vi "Log_Current_row_to_Execute.vi"(0 "Simulate/Run":T4, 1 "Message":string, 2 "Start of Multi Run Prog":bool, 3 "Traverse line in":T1 {"Carrier_2 Q (l/min)" format="%#.2f"; "Row Duration (mins)" format="%#.1f"; "Row No" min=0; "Trace Gas Concentration (%)" min=0.0 format="%#_4f"; "Carrier_1 Q (l/min)" format="%#.4f"; "Start X" format="%#.2f"; "Start Y" format="%#.2f"; "Start Z" format="%#.2f"; "End X" format="%#.2f"; "End Y" format="%#.2f"; "End Z" format="%#.2f"; "Tunnel Speed" format="%#.2f"; "Averaging time (mins)" min=0.0 format="%#.2f"}, 4 "Multi Run Log File":path) -> (9 "Traverse line Out":T1 {"Carrier_2 Q (l/min)" format="%#.2f"; "Row Duration (mins)" format="%#.1f"; "Row No" min=0; "Trace Gas Concentration (%)" min=0.0 format="%#_4f"; "Carrier_1 Q (l/min)" format="%#.4f"; "Start X" format="%#.2f"; "Start Y" format="%#.2f"; "Start Z" format="%#.2f"; "End X" format="%#.2f"; "End Y" format="%#.2f"; "End Z" format="%#.2f"; "Tunnel Speed" format="%#.2f"; "Averaging time (mins)" min=0.0 format="%#.2f"})   [LabVIEW 2020]
uses:
  Traverse_cluster.ctl
  Spacing.ctl
  Controls/Multi_run_mode.ctl
  Controls/User_Specific_mode.ctl
  Controls/Overhead.ctl
  Globals/Trav_pos_global.vi
panel:
  # "X                Y                   Z"
  # "X           Y          Z"
  # "Start"
  # "End"
  # "X           Y          Z"
  # "Start"
  # "End"
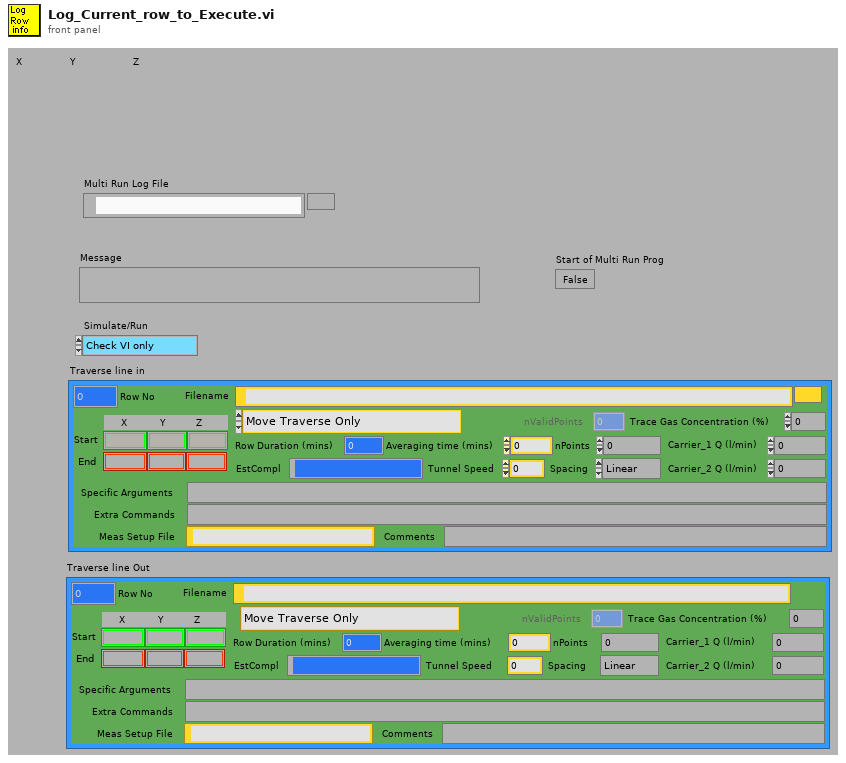
[diagram p1: front panel]
types:
  T1 = typedef "Traverse_cluster.ctl" = cluster{"Start X":sgl, "Start Y":sgl, "Start Z":sgl, "End X":sgl, "End Y":sgl, "End Z":sgl, "nPoints":i32, "Spacing":T2, "Filename":path, "Tunnel Speed":dbl, "Averaging time (mins)":dbl, "Extra Commands":string, "Carrier_1 Q (l/min)":dbl, "Carrier_2 Q (l/min)":dbl, "Trace Gas Concentration (%)":dbl, "Specific Arguments":string, "Comments":string, "Row No":i32, "Row Type Selector":T3, "EstCompl":string, "Row Duration (mins)":dbl, "nValidPoints":i32, "Meas Setup File":string}
  T2 = typedef "Spacing.ctl" = enum16{"Linear", "Log", "Gauss", "Specified", "N/A"}
  T3 = typedef "Multi_run_mode.ctl" = enum16{"Move Traverse Only", "Set Tunnel Speed Only", "Set Source Only", "Set Measurement Conditions", "Single Measurement", "Vertical Profile", "Lateral Profile", "Longitudinal Profile", "Multi-Axis Profile", "Explore Volume", "Auto Calibrate", "Meas Fast FID Bkgnd", "Check Beam Power", "Scanning Valve Measurement", "Run VI Named:", "Set ADAM Ch", "Wait (minutes)", "Send Message", "Synchronize With:", "Fall Back to this Row", "Turn Off Row Repeating", "Traverse 3D Volume", "Blank Row", "Jump to Fall Back Row"}
  T4 = typedef "User_Specific_mode.ctl" = enum16{"Check VI only", "Run VI"}
  T5 = enum16{"All Channel Names", "Valid Channel Names"}
  T6 = typedef "Overhead.ctl" = enum16{"Update total times", "Read Current Overhead", "Re Scale totals to 3 hrs", "Initialise totals to 3hr"}
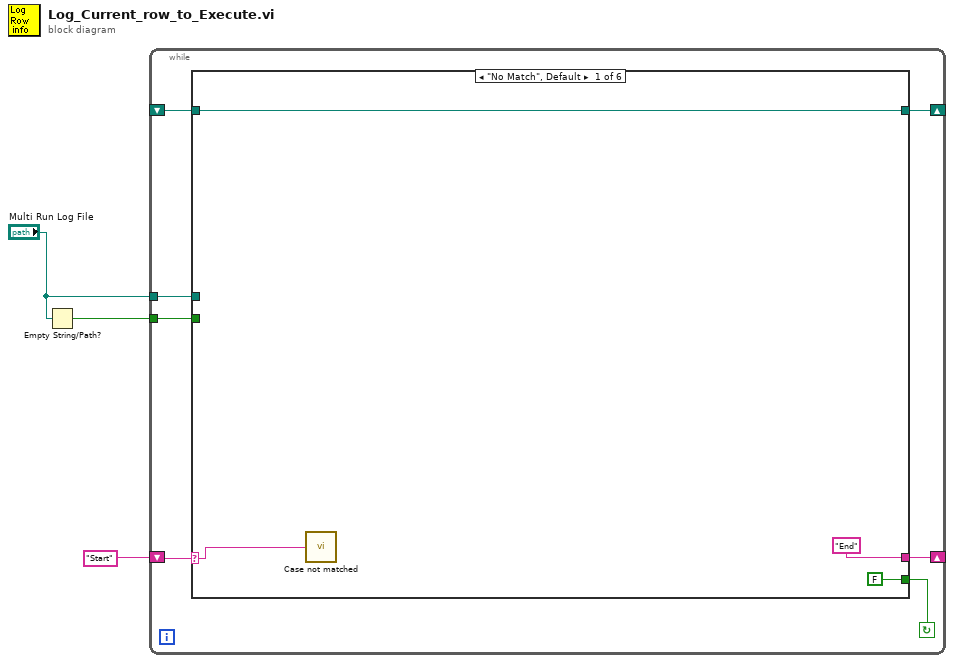
[diagram p0: block diagram]
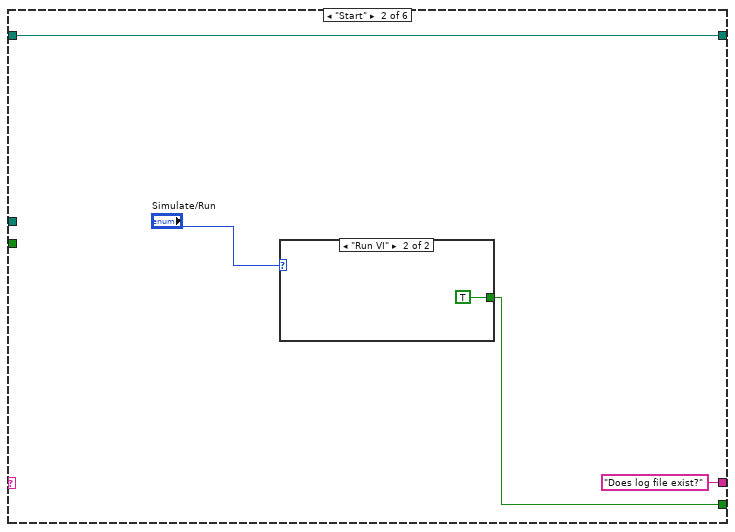
[diagram p2: hidden frame]
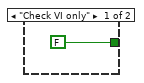
[diagram p3: hidden frame]
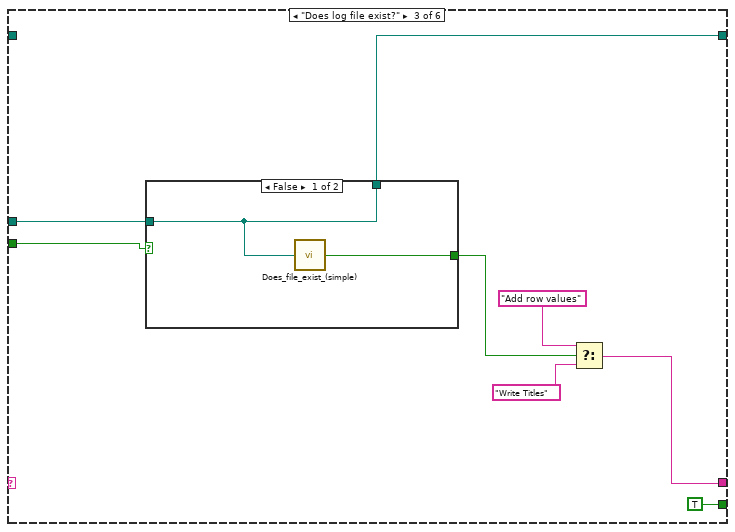
[diagram p4: hidden frame]
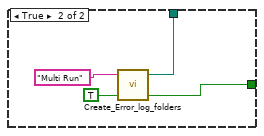
[diagram p5: hidden frame]
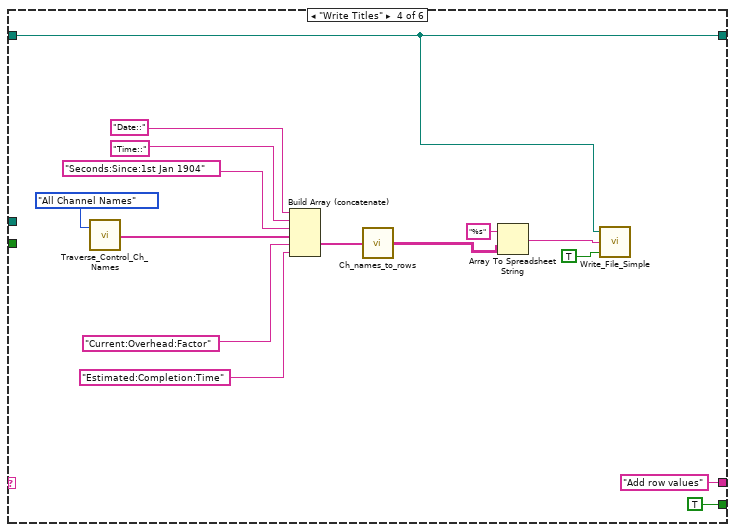
[diagram p6: hidden frame]
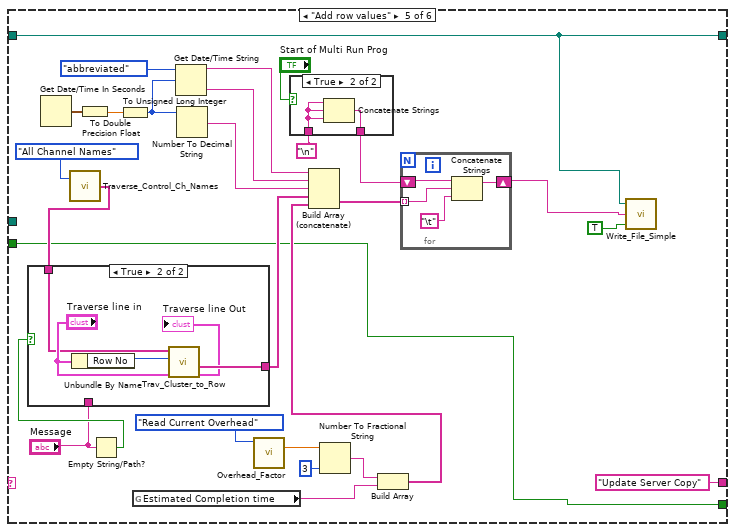
[diagram p7: hidden frame]
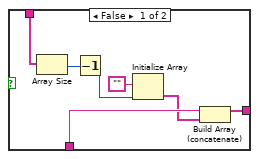
[diagram p9: hidden frame]
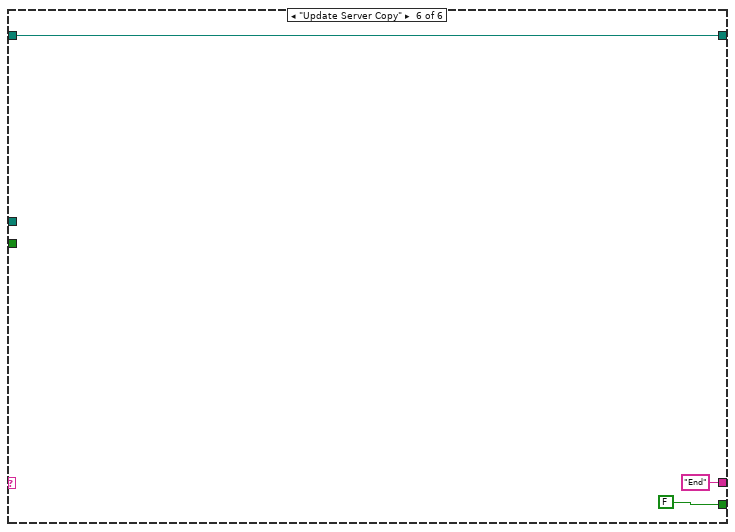
[diagram p10: hidden frame]
diagram:
  n1 = Empty String/Path?(string/path="Multi Run Log File") -> (empty?=w1:bool)
  n2 = while {
    shift-left: _ -> [w7]
    shift-right: [w8] -> _
    shift-left: "Start" -> [w6]
    shift-right: [w9] -> _
    tunnel: "Multi Run Log File" -> [w5]
    tunnel: w1 -> [w4]
    stop <- w10 continue-if-true
    n3 = case shown="\"No Match\", Default" w6 {
      selector: w6 -> [w11 _ _ _ _ _]
      tunnel: [FALSE ("T button?") w16 TRUE ("T button?") TRUE ("T button?") w53 FALSE] -> w10
      tunnel: ["End" "Does log file exist?" w28 "Add row values" "Update Server Copy" "End" ("f")] -> w9
      tunnel: [w12 w18 w26 w35 w50 w96] -> w8
      tunnel: w7 -> [w12 w18 _ w35 w50 w96]
      tunnel: w5 -> [_ _ w22 _ _ _]
      tunnel: w4 -> [_ _ w21 _ w53 _]
      frame "No Match", Default {
        n4 = call "Case not matched.vi"("Case Name not Matched"=w11) -> ()
      }
      frame "Start" {
        n5 = case shown="\"Run VI\"" "Simulate/Run" {
          tunnel: [FALSE TRUE] -> w16
          frame "Check VI only" {
          }
          frame "Run VI" {
          }
        }
      }
      frame "Does log file exist?" {
        n6 = case shown="False" w21 {
          tunnel: [w30 w34] -> w26
          tunnel: [w29 w32] -> w25
          tunnel: w22 -> [w30 _]
          frame False {
            n7 = call "Does_file_exist_(simple).vi"("Pathname"=w30) -> ("exists?"=w29:bool)
          }
          frame True {
            n8 = call "Create_Error_log_folders.vi"("Log Filename"="Multi Run" ("Input Element"), "Per Day Log File?"=TRUE) -> ("Local Log File"=w34:path, "exists?"=w32:bool)  [unwired: 4 in]
          }
        }
        n9 = Select(t="Add row values", s=w25, f="Write Titles") -> (s? t:f=w28:string)
      }
      frame "Write Titles" {
        n10 = call "Traverse_Control_Ch_Names.vi"("Mode"=T5."All Channel Names") -> ("Channel names"=w43:string[])  [unwired: 1 in]
        n11 = Build Array (concatenate)("Date::", "Time::", "Seconds:Since:1st Jan 1904", w43, "Current:Overhead:Factor", "Estimated:Completion:Time") -> (w40:string[])
        n12 = call "Ch_names_to_rows.vi"("Channel Names"=w40) -> ("3 Row names"=w39:string[][])
        n13 = Array To Spreadsheet String(array=w39, 3:"%s" ("format string")) -> (spreadsheet string=w36:string)  [unwired: 1 out]
        n14 = call "Write_File_Simple.vi"("append to file? (new file:F)"=TRUE, "character string"=w36, "file path"=w35) -> ()  [unwired: 2 out]
      }
      frame "Add row values" {
        n15 = Get Date/Time In Seconds() -> (seconds since 1Jan1904=w54:timestamp)
        n16 = call "Traverse_Control_Ch_Names.vi"("Mode"=T5."All Channel Names") -> ("Channel names"=w66:string[])  [unwired: 1 in]
        n17 = To Double Precision Float(number=w54) -> (double precision float=w75:dbl)
        n18 = Empty String/Path?(string/path="Message") -> (empty?=w68:bool)
        n19 = case shown="True" w68 {
          tunnel: w66 -> [w85 w89]
          tunnel: [w83 w88] -> w70
          tunnel: "Message" -> [w86 _]
          frame False {
            n20 = Array Size(array=w85) -> (size(s)=w82:i32)
            n21 = Decrement(x=w82) -> (x-1=w81:i32)
            n22 = Initialize Array("", w81) -> (w80:string[])
            n23 = Build Array (concatenate)(w86, w80) -> (w83:string[])
          }
          frame True {
            n24 = Unbundle By Name("Traverse line in") -> ("Row No"=w91:i32)
            n25 = call "Trav_Cluster_to_Row.vi"("Traverse line in"="Traverse line in", "Row Number"=w91, "Channel names"=w89) -> ("Traverse line Out"=→"Traverse line Out":T1, "Channel Values Out"=w88:string[])  [unwired: 3 out]
          }
        }
        n26 = To Unsigned Long Integer(number=w75) -> (unsigned 32bit integer=w76:u32)
        n27 = global read "Trav_pos_global.vi" "Estimated Completion time"() -> (w63:string)
        n28 = Get Date/Time String(date format (0)=enum16{"short", "long", "abbreviated"}."abbreviated", seconds (now)=w76) -> (date string=w74:string, time string=w73:string)  [unwired: 1 out]
        n29 = Number To Decimal String(number=w76) -> (decimal integer string=w72:string)  [unwired: 1 out]
        n30 = call "Overhead_Factor.vi"("Mode"=Overhead."Read Current Overhead") -> ("Current Overhead Factor"=w56:dbl)  [unwired: 3 in]
        n31 = case shown="True" "Start of Multi Run Prog" {
          tunnel: [w77 w79] -> w59
          tunnel: "\n" -> [w77 w78]
          frame False {
          }
          frame True {
            n32 = Concatenate Strings(w78, w78, w78) -> (w79:string)
          }
        }
        n33 = Number To Fractional String(number=w56, precision (6)=i16 3) -> (F-format string=w64:string)  [unwired: 2 out]
        n34 = Build Array(w64, w63) -> (w62:string[])
        n35 = Build Array (concatenate)(w74, w73, w72, w70, w62) -> (w71:string[])
        n36 = for {
          shift-right: [w94] -> w51
          shift-left: w59 -> [w95]
          tunnel: w71 -> [w93] mode=indexing
          n37 = Concatenate Strings(w95, w93, "\t") -> (w94:string)
        }
        n38 = call "Write_File_Simple.vi"("append to file? (new file:F)"=TRUE, "character string"=w51, "file path"=w50) -> ()  [unwired: 2 out]
      }
      frame "Update Server Copy" {
      }
    }
  }
